vi "Bed_control.vi"(8 "Motor speed":string(combo)="Full step", 9 "pulse duration (T/2)":dbl=0.0005 format="%#_13p", 10 "Sequence to run on start up":string[](array[string]), 11 "Signed pulses to move":dbl=50.0) -> ()   [LabVIEW 2021]
uses:
  <vilib>/DAQmx/write.llb/DAQmx Write (Digital 1D Wfm NChan NSamp).vi
  <vilib>/DAQmx/read.llb/DAQmx Read (Digital 1D Bool 1Chan 1Samp).vi
  <vilib>/Waveform/DWDTOps.llb/DWDT Digital Size.vi
  SmallBore_Labview/global_variables.vi
  <vilib>/DAQmx/create/channels.llb/DAQmx Create Channel (DO-Digital Output).vi
  <vilib>/DAQmx/configure/timing.llb/DAQmx Timing (Sample Clock).vi
  <vilib>/Waveform/DWDTOps.llb/DWDT Uncompress Digital.vi
  <vilib>/DAQmx/miscellaneous.llb/DAQmx Fill In Error Info.vi
  <vilib>/DAQmx/create/channels.llb/DAQmx Create Channel (DI-Digital Input).vi
panel:
  out "data":bool[](array[boolean])
  out "Bed latch switch lines":tag="Dev1/port0/line5:6"
  out "x-y":dbl=626.4
  out "-x":dbl=-24.1
  out "Slide":dbl(slide) min=-35.9 max=609.1 scale=-12.9..637.6
  out "Laser:End dist":dbl=626.4
  out "Home:End dist":dbl=650.5
  out "Home:Laser dist":dbl=24.1
  in  "Save Home-Laser Dist":bool
  in  "Enable Homing Interrupt":bool=TRUE
  in  "Sweep":bool
  out "Main loop has stopped":bool
  out "Last system state called":string="Move"
  in  "Read position":bool
  out "Boolean":bool=TRUE
  in  "Number of runs (>1)":i32=3
  out "Bed position":dbl
  out "Application Directory":path=path "C:/Users/MPI/Documents/GitHub/LabviewGUI"
  out "travel distance (mm)":dbl=5.0
  in  "pulse steps":dbl=50.0 min=0.0 step=1.0 format="%#_6p"
  in  "Move bed 2":bool
  out "Homing in progress":bool
  out "duration of movement":dbl=0.05
  in  "Maximum absolute position":i32=60000 format="%.0p"
  out "Absolute position (pulses)":i32=13150
  in  "Abort movement":bool
  in  "Go home!":bool
  in  "Move bed":bool
  in  "Halt":bool
  # "For programatical use only!\nEnsure that the sequence control is empty before setting default values!"
  # "Step 1: Initiate Homing\nStep 2: Physically press ZERO button\nStep 3: Read position\nStep 4: Go to laser position\nStep 5: Read position\nStep 6: Save current position = Laser\nStep 7: Physically press ZERO button"
  # "Homing"
  # "Enables PDU automatically"
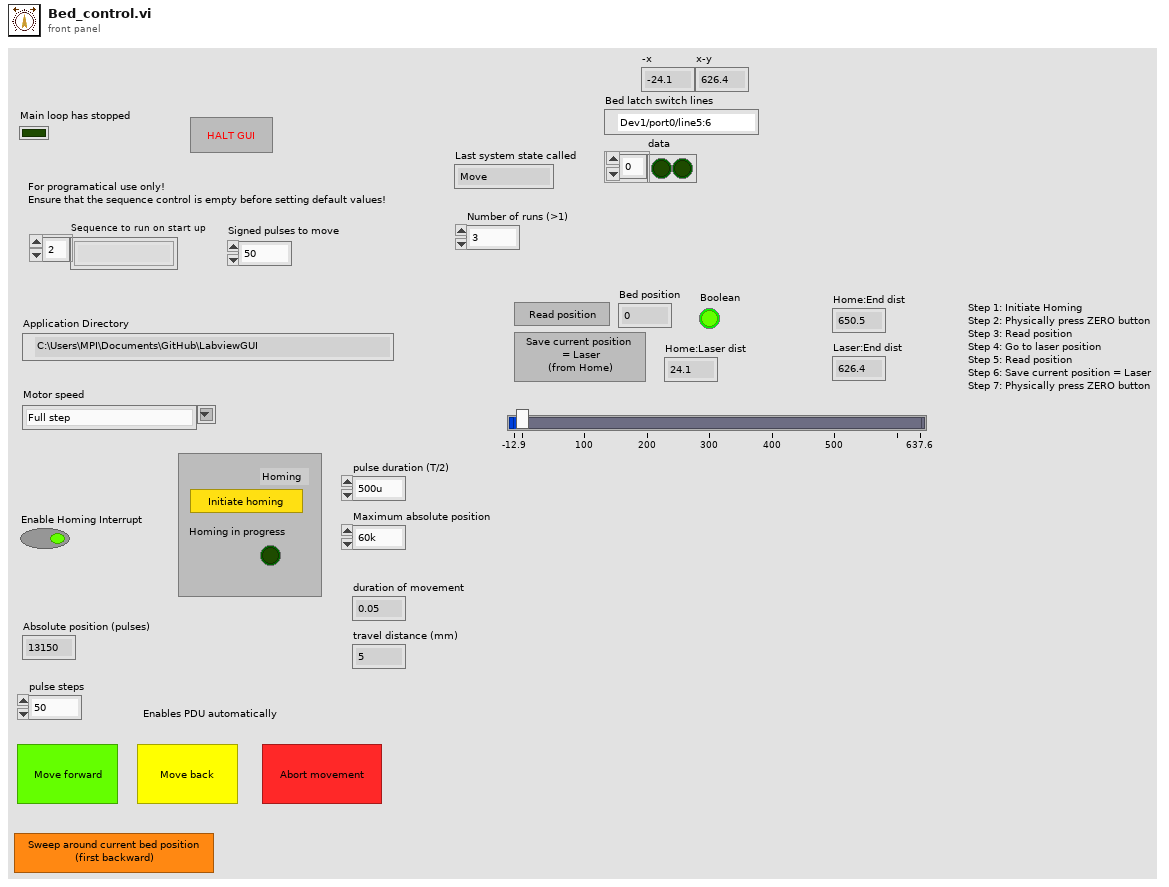
[diagram p1: front panel]
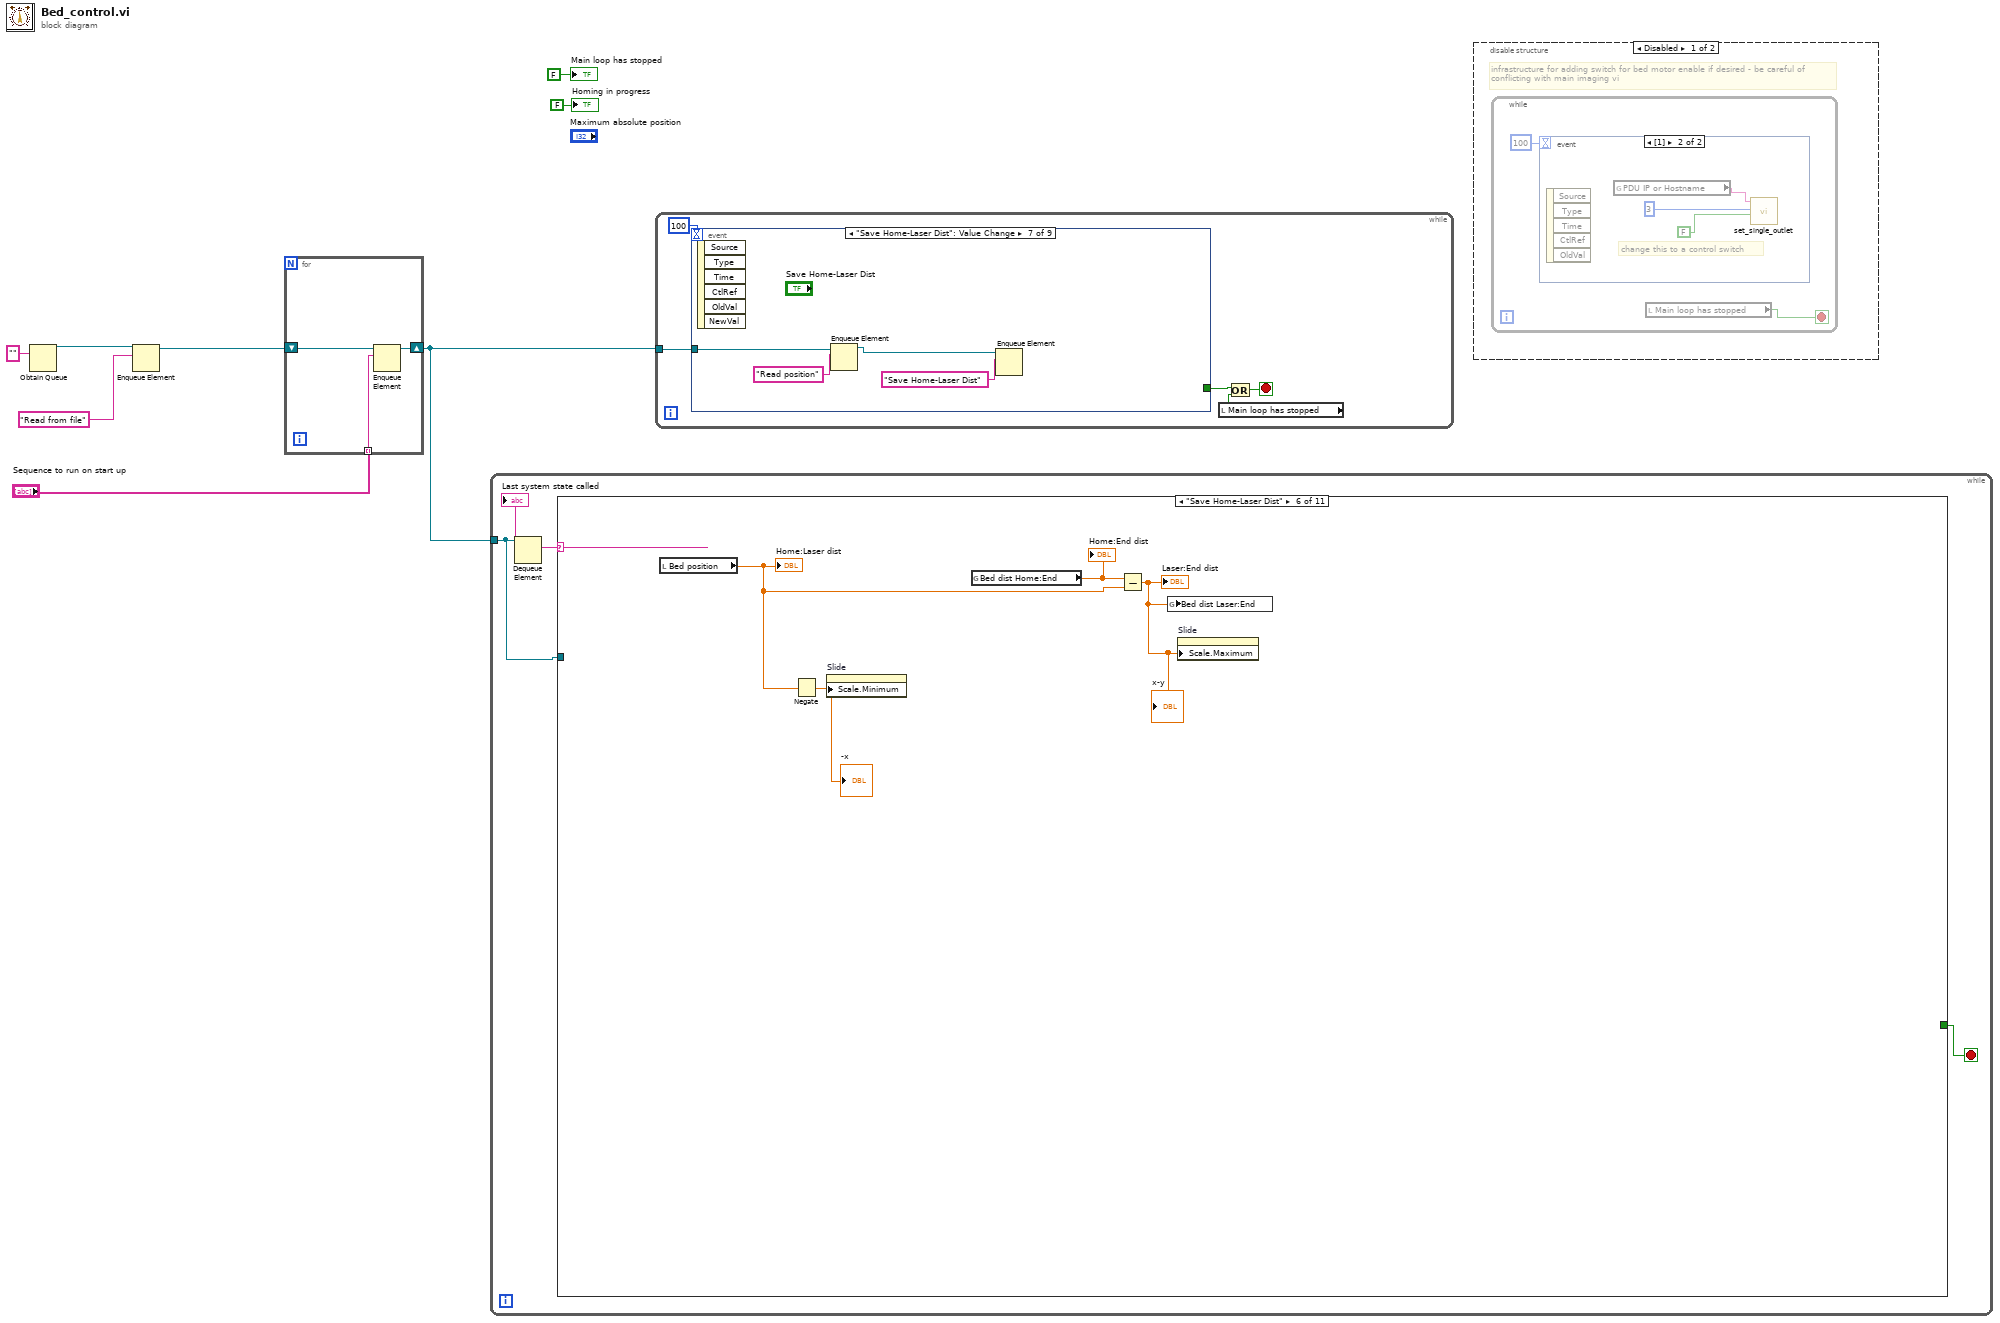
[diagram p0: block diagram]
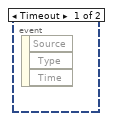
[diagram p2: hidden frame]
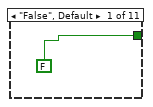
[diagram p4: hidden frame]
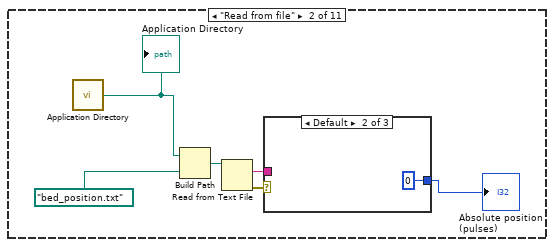
[diagram p5: hidden frame]
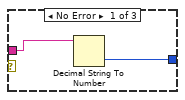
[diagram p6: hidden frame]
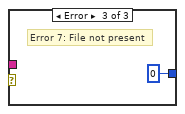
[diagram p7: hidden frame]
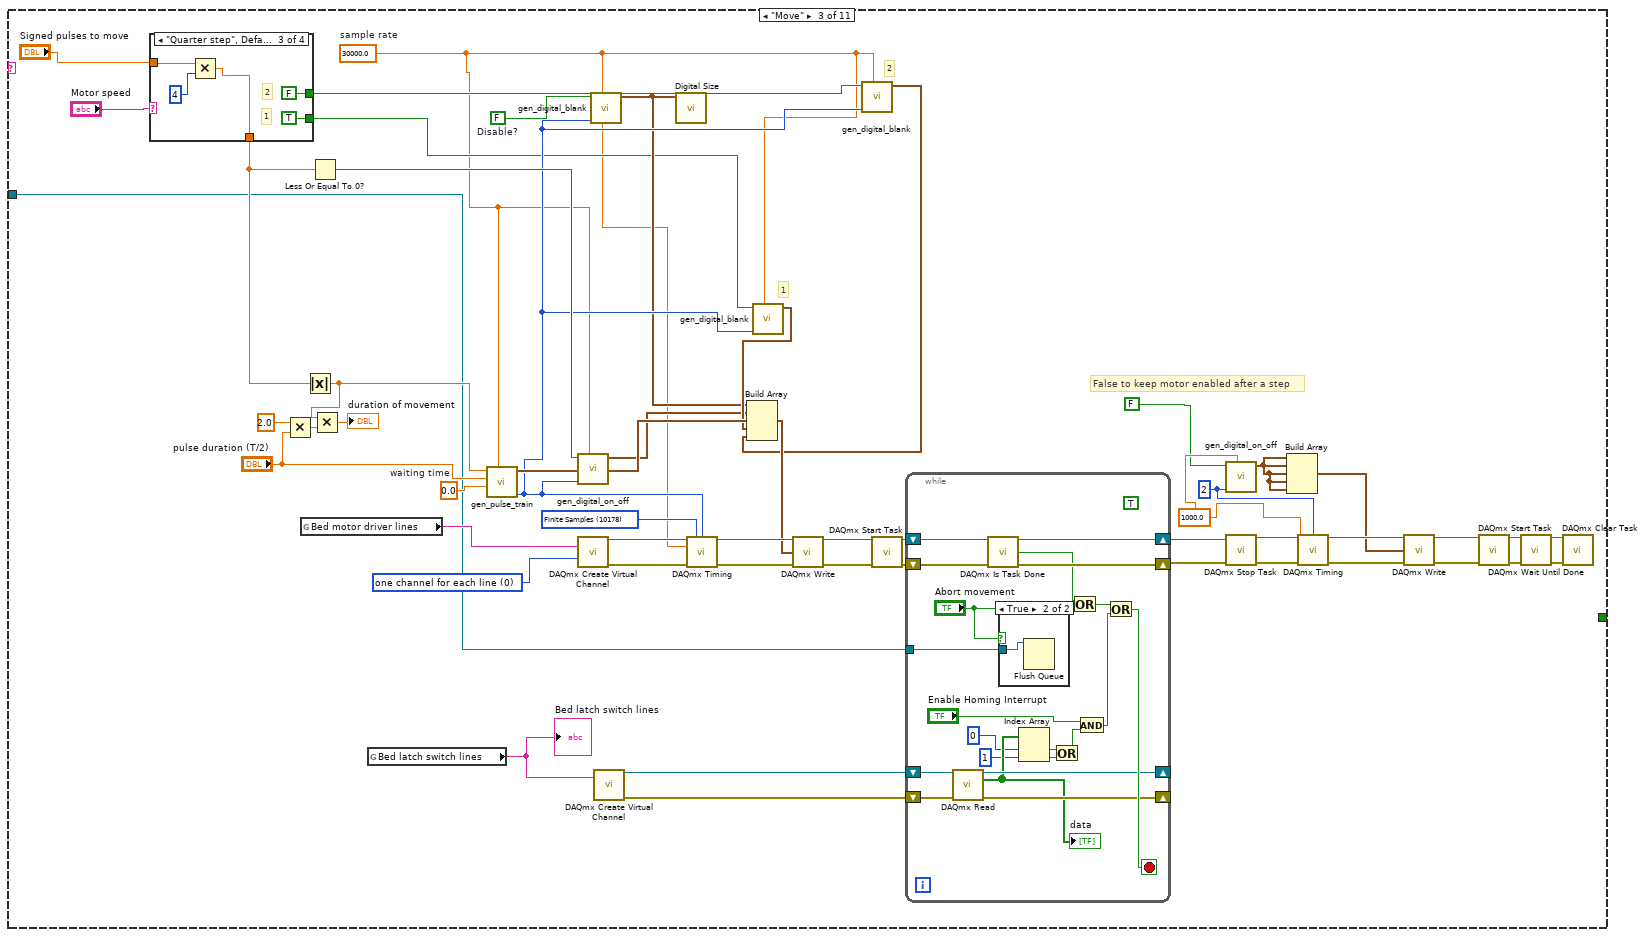
[diagram p8: hidden frame]
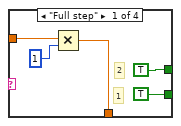
[diagram p9: hidden frame]
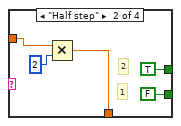
[diagram p10: hidden frame]
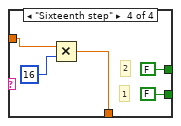
[diagram p11: hidden frame]
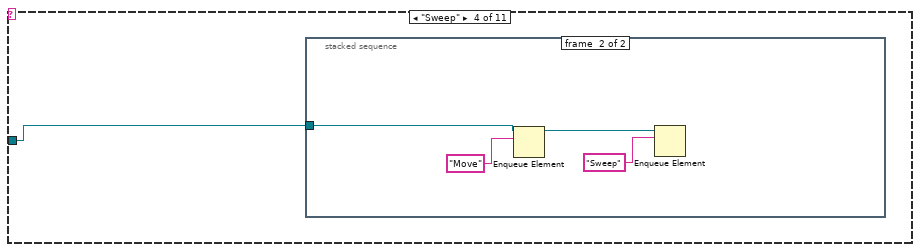
[diagram p13: hidden frame]
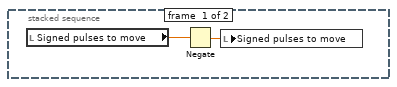
[diagram p14: hidden frame]
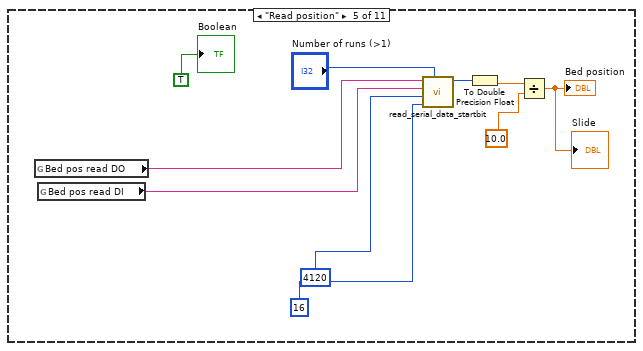
[diagram p15: hidden frame]
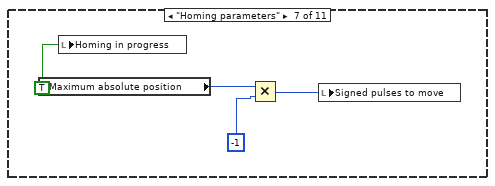
[diagram p16: hidden frame]
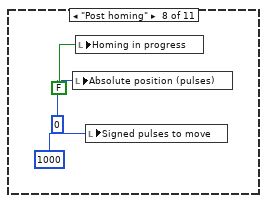
[diagram p17: hidden frame]
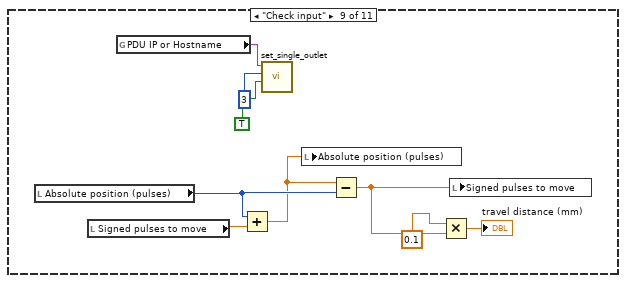
[diagram p18: hidden frame]
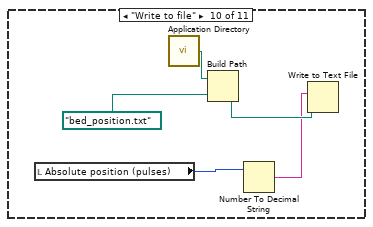
[diagram p19: hidden frame]
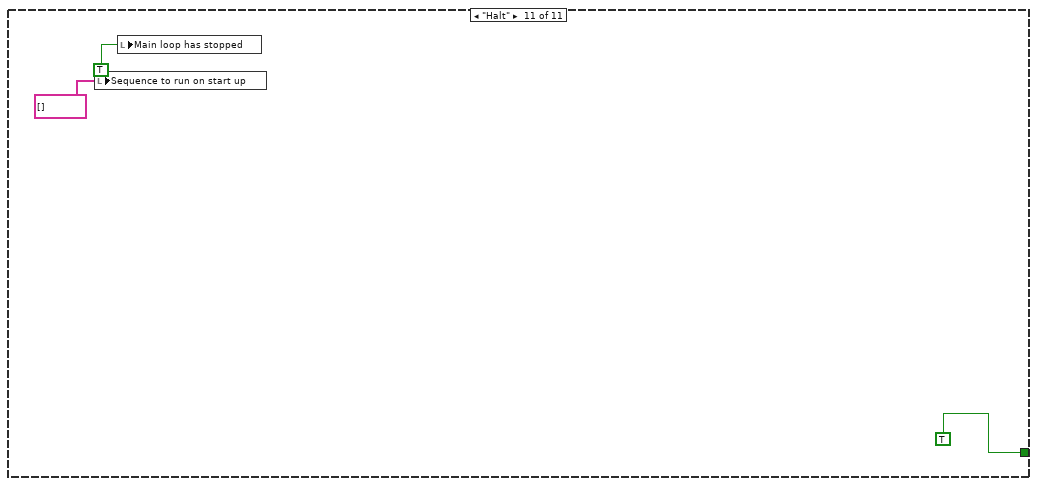
[diagram p20: hidden frame]
diagram:
  n1 = Obtain Queue(element data type="") -> (queue out=w7:refnum<queue>)  [unwired: 4 in, 2 out]
  n2 = Enqueue Element(queue=w7, element="Read from file") -> (queue out=w4:refnum<queue>)  [unwired: 2 in, 2 out]
  n3 = for {
    shift-right: [w10] -> w3
    shift-left: w4 -> [w11]
    tunnel: "Sequence to run on start up" -> [w9] mode=indexing
    n4 = Enqueue Element(queue=w11, element=w9) -> (queue out=w10:refnum<queue>)  [unwired: 2 in, 2 out]
  }
  n5 = while {
    tunnel: w3 -> [w12]
    stop <- w13 stop-if-true
    n6 = Dequeue Element(queue=w12) -> (element=w14:string)  [unwired: 2 in, 3 out]
    "Last system state called" <- w14
    n7 = case shown="\"Save Home-Laser Dist\"" w14 {
      tunnel: [FALSE _ _ _ _ _ _ _ _ _ TRUE] -> w13
      tunnel: w12 -> [_ _ w29 w121 _ _ _ _ _ _ _]
      frame "False", Default {
      }
      frame "Read from file" {
        n8 = call <vilib>:"Application Directory.vi"() -> ("Application Directory"=w18:path)
        "Application Directory" <- w18
        n9 = Build Path(base path=w18, name or relative path=path "bed_position.txt" ("file (use dialog)")) -> (appended path=w19:path)
        n10 = Read from Text File(file (use dialog)=w19) -> (text=w21:string, error out=w20:errorcluster)  [unwired: 3 in, 2 out]
        n11 = case shown="Default" w20 {
          tunnel: w21 -> [w23 _ _]
          tunnel: [w22 0 0] -> w16
          frame No Error {
            n12 = Decimal String To Number(string=w23) -> (number=w22:i32)  [unwired: 2 in, 1 out]
          }
          frame Default {
          }
          frame Error {
            # "Error 7: File not present"
          }
        }
        "Absolute position (pulses)" <- w16
      }
      frame "Move" {
        w45 = 2 ("waveform length")
        w46 = 1000.0 ("rate")
        w68 = 0.0  # waiting time
        w28 = 30000.0  # sample rate
        w71 = FALSE  # Disable?
        w70 = 10178 items=["Finite Samples"=10178, "Continuous Samples"=10123, "Hardware Timed Single Point"=12522] ("sample mode")
        w69 = 0 items=["one channel for each line", "one channel for all lines"] ("line grouping")
        # "1"
        # "2"
        # "False to keep motor enabled after a step"
        n13 = case shown="\"Quarter step\", Default" "Motor speed" {
          tunnel: "Signed pulses to move" -> [w82 w87 w92 w97]
          tunnel: [TRUE ("motor speed control 1") TRUE ("motor speed control 1") FALSE ("motor speed control 1") FALSE ("motor speed control 1")] -> w35
          tunnel: [TRUE ("motor speed control 1") FALSE ("motor speed control 1") TRUE ("motor speed control 1") FALSE ("motor speed control 1")] -> w34
          tunnel: [w79 w84 w89 w94] -> w33
          frame "Full step" {
            # "1"
            # "2"
            n14 = Multiply(x=w82, y=1) -> (x*y=w79:dbl)
          }
          frame "Half step" {
            # "1"
            # "2"
            n15 = Multiply(x=w87, y=2) -> (x*y=w84:dbl)
          }
          frame "Quarter step", Default {
            # "1"
            # "2"
            n16 = Multiply(x=w92, y=4) -> (x*y=w89:dbl)
          }
          frame "Sixteenth step" {
            # "1"
            # "2"
            n17 = Multiply(x=w97, y=16) -> (x*y=w94:dbl)
          }
        }
        n18 = Multiply(x=2.0, y="pulse duration (T/2)") -> (x*y=w64:dbl)
        n19 = global read "global_variables.vi" "Bed motor driver lines"() -> (w32:tag)
        n20 = Absolute Value(x=w33) -> (abs(x)=w65:dbl)
        n21 = Less Or Equal To 0?(x=w33) -> (x <= 0?=w67:bool)
        n22 = Multiply(x=w65, y=w64) -> (x*y=→"duration of movement":dbl)
        n23 = global read "global_variables.vi" "Bed latch switch lines"() -> (w31:tag)
        "Bed latch switch lines" <- w31
        n24 = call "gen_pulse_train.vi"("sampling rate"=w28, "waiting time"=w68, "pulse width"="pulse duration (T/2)", "Number of pulses"=w65) -> ("waveform length"=w42:i32, "digital waveform out"=w76:digitalwaveform)  [unwired: 6 in]
        n25 = call "gen_digital_on_off.vi"("sampling rate"=w28, "waveform length"=w42, "On / Off"=w67) -> ("digital waveform"=w37:digitalwaveform)  [unwired: 8 in]
        n26 = call-poly <vilib>:"DAQmx Create Virtual Channel.vi"("lines"=w32, "line grouping"=w69) -> ("task out"=w72:refnum<k21>, "error out"=w75:errorcluster)  [unwired: 12 in]
        n27 = call "gen_digital_blank.vi"("sampling rate"=w28, "waveform length"=w42, "On / Off"=w71) -> ("digital waveform"=w38:digitalwaveform)  [unwired: 8 in]
        n28 = call-poly <vilib>:"DAQmx Create Virtual Channel.vi"("lines"=w31) -> ("task out"=w27:refnum<k21>, "error out"=w26:errorcluster)  [unwired: 13 in]
        n29 = call-poly <vilib>:"Digital Size.vi"("digital waveform in"=w38) -> ()  [unwired: 7 in, 4 out]
        n30 = call-poly <vilib>:"DAQmx Timing.vi"("task/channels in"=w72, "sample mode"=w70, "samples per channel"=w42, "rate"=w28, "error in"=w75) -> ("task out"=w73:refnum<k21>, "error out"=w74:errorcluster)  [unwired: 9 in]
        n31 = call "gen_digital_blank.vi"("sampling rate"=w28, "waveform length"=w42, "On / Off"=w34) -> ("digital waveform"=w39:digitalwaveform)  [unwired: 8 in]
        n32 = call "gen_digital_blank.vi"("sampling rate"=w28, "waveform length"=w42, "On / Off"=w35) -> ("digital waveform"=w40:digitalwaveform)  [unwired: 8 in]
        n33 = Build Array(w38, w37, w76, w39, w40) -> (w44:digitalwaveform[])
        n34 = call-poly <vilib>:"DAQmx Write.vi"("task/channels in"=w73, "data"=w44, "error in"=w74) -> ("task out"=w77:refnum<k21>, "error out"=w78:errorcluster)  [unwired: 10 in, 1 out]
        n35 = call <vilib>:"DAQmx Start Task.vi"("task/channels in"=w77, "error in"=w78) -> ("task out"=w61:refnum<k21>, "error out"=w60:errorcluster)  [unwired: 12 in]
        n36 = while {
          shift-right: [w116] -> w58
          shift-left: w60 -> [w118]
          shift-right: [w117] -> w59
          shift-left: w61 -> [w119]
          shift-right: [w109] -> _
          shift-left: w27 -> [w112]
          shift-right: [w110] -> _
          shift-left: w26 -> [w111]
          tunnel: w29 -> [w107]
          stop <- w113 stop-if-true
          (unwired) TRUE ("Abort movement")
          n37 = call-poly <vilib>:"DAQmx Read.vi"("task/channels in"=w112, "error in"=w111) -> ("task out"=w109:refnum<k21>, "data"=w104:bool[], "error out"=w110:errorcluster)  [unwired: 11 in]
          "data" <- w104
          n38 = call <vilib>:"DAQmx Is Task Done.vi"("task/channels in"=w119, "error in"=w118) -> ("task out"=w117:refnum<k21>, "task done?"=w115:bool, "error out"=w116:errorcluster)  [unwired: 11 in]
          n39 = case shown="True" "Abort movement" {
            tunnel: w107 -> [_ w120]
            frame False {
            }
            frame True {
              n40 = Flush Queue(queue=w120) -> ()  [unwired: 1 in, 3 out]
            }
          }
          n41 = Index Array(array=w104, index #1=0 ("index"), index #2=1 ("index")) -> (element #1=w100:bool, element #2=w99:bool)
          n42 = Or(x=w100, y=w99) -> (x .or. y?=w101:bool)
          n43 = Or(x=w115, y="Abort movement") -> (x .or. y?=w114:bool)
          n44 = And(x="Enable Homing Interrupt", y=w101) -> (x .and. y?=w105:bool)
          n45 = Or(x=w114, y=w105) -> (x .or. y?=w113:bool)
        }
        n46 = call "gen_digital_on_off.vi"("sampling rate"=w46, "waveform length"=w45, "On / Off"=FALSE ("Keep enabled\n(inverted logic)")) -> ("digital waveform"=w41:digitalwaveform)  [unwired: 8 in]
        n47 = call <vilib>:"DAQmx Stop Task.vi"("task/channels in"=w59, "error in"=w58) -> ("task out"=w48:refnum<k21>, "error out"=w51:errorcluster)  [unwired: 12 in]
        n48 = Build Array(w41, w41, w41, w41, w41) -> (w47:digitalwaveform[])
        n49 = call-poly <vilib>:"DAQmx Timing.vi"("task/channels in"=w48, "samples per channel"=w45, "rate"=w46, "error in"=w51) -> ("task out"=w49:refnum<k21>, "error out"=w50:errorcluster)  [unwired: 10 in]
        n50 = call-poly <vilib>:"DAQmx Write.vi"("task/channels in"=w49, "data"=w47, "error in"=w50) -> ("task out"=w57:refnum<k21>, "error out"=w56:errorcluster)  [unwired: 10 in, 1 out]
        n51 = call <vilib>:"DAQmx Start Task.vi"("task/channels in"=w57, "error in"=w56) -> ("task out"=w55:refnum<k21>, "error out"=w54:errorcluster)  [unwired: 12 in]
        n52 = call <vilib>:"DAQmx Wait Until Done.vi"("task/channels in"=w55, "error in"=w54) -> ("task out"=w53:refnum<k21>, "error out"=w52:errorcluster)  [unwired: 12 in]
        n53 = call <vilib>:"DAQmx Clear Task.vi"("task in"=w53, "error in"=w52) -> ()  [unwired: 13 in, 1 out]
      }
      frame "Sweep" {
        n54 = stacked-sequence {
          tunnel: w121 -> [_ w126]
          frame #0 {
            n55 = local read "Signed pulses to move"() -> (w123:dbl)
            n56 = Negate(x=w123) -> (-x=w122:dbl)
            n57 = local write "Signed pulses to move"(w122) -> ()
          }
          frame #1 {
            n58 = Enqueue Element(queue=w126, element="Move") -> (queue out=w124:refnum<queue>)  [unwired: 2 in, 2 out]
            n59 = Enqueue Element(queue=w124, element="Sweep") -> ()  [unwired: 2 in, 3 out]
          }
        }
      }
      frame "Read position" {
        n60 = global read "global_variables.vi" "Bed pos read DO"() -> (w132:tag)
        n61 = global read "global_variables.vi" "Bed pos read DI"() -> (w131:tag)
        n62 = call "read_serial_data_startbit.vi"("Number of runs"="Number of runs (>1)", "No. expected bits"=u16 16, "baud rate"=u32 4120, "Digital input line"=w131, "Digital output line"=w132) -> ("mode"=w137:i16)  [unwired: 4 in, 1 out]
        n63 = To Double Precision Float(number=w137) -> (double precision float=w135:dbl)
        n64 = Divide(x=w135, y=10.0) -> (x/y=→"Bed position" →"Slide":dbl)
        "Boolean" <- TRUE ("Boolean")
      }
      frame "Save Home-Laser Dist" {
        n65 = local read "Bed position"() -> (w140:dbl)
        "Home:Laser dist" <- w140
        n66 = Negate(x=w140) -> (-x=w139:dbl)
        "-x" <- w139
        n67 = property on="Slide" class="Slide (strict)"("Scale.Minimum"=w139) -> ()  [unwired: 2 in, 2 out]
        n68 = global read "global_variables.vi" "Bed dist Home:End"() -> (w141:dbl)
        "Home:End dist" <- w141
        n69 = Subtract(x=w141, y=w140) -> (x-y=w138:dbl)
        "Laser:End dist" <- w138
        "x-y" <- w138
        n70 = global write "global_variables.vi" "Bed dist Laser:End"(w138) -> ()
        n71 = property on="Slide" class="Slide (strict)"("Scale.Maximum"=w138) -> ()  [unwired: 2 in, 2 out]
      }
      frame "Homing parameters" {
        n72 = local read "Maximum absolute position"() -> (w144:i32)
        n73 = local write "Homing in progress"(TRUE ("Homing in progress")) -> ()
        n74 = Multiply(x=w144, y=-1) -> (x*y=w142:i32)
        n75 = local write "Signed pulses to move"(w142) -> ()
      }
      frame "Post homing" {
        n76 = local write "Absolute position (pulses)"(0 ("Absolute position (pulses)")) -> ()
        n77 = local write "Homing in progress"(FALSE ("Homing in progress")) -> ()
        n78 = local write "Signed pulses to move"(1000 ("pulses to move")) -> ()
      }
      frame "Check input" {
        n79 = local read "Absolute position (pulses)"() -> (w157:i32)
        n80 = local read "Signed pulses to move"() -> (w150:dbl)
        n81 = global read "global_variables.vi" "PDU IP or Hostname"() -> (w153:string)
        n82 = Add(x=w157, y=w150) -> (x+y=w149:dbl)
        n83 = call "set_single_outlet.vi"("Switch state"=TRUE, "Outlet #"=3, "IP / Hostname"=w153) -> ()  [unwired: 9 in]
        n84 = local write "Absolute position (pulses)"(w149) -> ()
        n85 = Subtract(x=w149, y=w157) -> (x-y=w154:dbl)
        n86 = Multiply(x=0.1, y=w154) -> (x*y=→"travel distance (mm)":dbl)
        n87 = local write "Signed pulses to move"(w154) -> ()
      }
      frame "Write to file" {
        n88 = local read "Absolute position (pulses)"() -> (w158:i32)
        n89 = call <vilib>:"Application Directory.vi"() -> ("Application Directory"=w162:path)
        n90 = Build Path(base path=w162, name or relative path=path "bed_position.txt" ("file (use dialog)")) -> (appended path=w161:path)
        n91 = Number To Decimal String(number=w158) -> (decimal integer string=w160:string)  [unwired: 1 in]
        n92 = Write to Text File(file (use dialog)=w161, text=w160) -> ()  [unwired: 2 in, 3 out]
      }
      frame "Halt" {
        n93 = local write "Sequence to run on start up"(string[] [] ("Sequence to run on start up")) -> ()
        n94 = local write "Main loop has stopped"(TRUE ("Main loop has stopped")) -> ()
      }
    }
  }
  n95 = while {
    tunnel: w3 -> [w170]
    stop <- w167 stop-if-true
    n96 = event shown="[6] \"Save Home-Laser Dist\": Value Change" {
      selector: _ -> [_ _ _ _ _ _ _ _ _]
      dyn-events: _ -> [_ _ _ _ _ _ _ _ _]
      timeout: 100 -> [_ _ _ _ _ _ _ _ _]
      tunnel: w170 -> [_ w174 w175 w181 _ w185 w194 w201 w204]
      tunnel: [FALSE TRUE _ _ _ _ _ _ _] -> w168
      event Timeout {
        n97 = event-data() -> ()  [unwired: 1 in, 3 out]
      }
      event "Halt": Value Change {
        n98 = event-data() -> ()  [unwired: 1 in, 6 out]
        n99 = Enqueue Element(queue=w174, element="Halt") -> ()  [unwired: 2 in, 3 out]
      }
      event "Move bed": Value Change {
        n100 = event-data() -> ()  [unwired: 1 in, 6 out]
        n101 = stacked-sequence {
          tunnel: w175 -> [_ w177]
          frame #0 {
            n102 = local write "Signed pulses to move"("pulse steps") -> ()
          }
          frame #1 {
            n103 = Enqueue Element(queue=w177, element="Check input") -> (queue out=w178:refnum<queue>)  [unwired: 2 in, 2 out]
            n104 = Enqueue Element(queue=w178, element="Move") -> ()  [unwired: 2 in, 3 out]
          }
        }
      }
      event "Sweep": Value Change {
        n105 = event-data() -> ()  [unwired: 1 in, 6 out]
        n106 = stacked-sequence {
          tunnel: w181 -> [_ w183]
          frame #0 {
            n107 = local read "pulse steps"() -> (w182:dbl)
            n108 = local write "Signed pulses to move"(w182) -> ()
          }
          frame #1 {
            n109 = Enqueue Element(queue=w183, element="Sweep") -> ()  [unwired: 2 in, 3 out]
          }
        }
      }
      event Key Down? {
        n110 = event-data() -> ()  [unwired: 1 in, 10 out]
        n111 = event-data() -> ()  [unwired: 7 in, 1 out]
      }
      event "Move bed 2": Value Change {
        n112 = event-data() -> ()  [unwired: 1 in, 6 out]
        n113 = stacked-sequence {
          tunnel: w185 -> [_ w188]
          frame #0 {
            n114 = local read "pulse steps"() -> (w186:dbl)
            n115 = Negate(x=w186) -> (-x=w187:dbl)
            n116 = local write "Signed pulses to move"(w187) -> ()
          }
          frame #1 {
            n117 = Enqueue Element(queue=w188, element="Check input") -> (queue out=w189:refnum<queue>)  [unwired: 2 in, 2 out]
            n118 = Enqueue Element(queue=w189, element="Move") -> ()  [unwired: 2 in, 3 out]
          }
        }
      }
      event "Save Home-Laser Dist": Value Change {
        n119 = event-data() -> ()  [unwired: 1 in, 6 out]
        n120 = Enqueue Element(queue=w194, element="Read position") -> (queue out=w192:refnum<queue>)  [unwired: 2 in, 2 out]
        n121 = Enqueue Element(queue=w192, element="Save Home-Laser Dist") -> ()  [unwired: 2 in, 3 out]
      }
      event "Go home!": Value Change {
        n122 = event-data() -> ()  [unwired: 1 in, 6 out]
        n123 = local write "Enable Homing Interrupt"("Go home!") -> ()
        n124 = Enqueue Element(queue=w201, element="Homing parameters") -> (queue out=w199:refnum<queue>)  [unwired: 2 in, 2 out]
        n125 = Enqueue Element(queue=w199, element="Move") -> (queue out=w197:refnum<queue>)  [unwired: 2 in, 2 out]
        n126 = Enqueue Element(queue=w197, element="Post homing") -> ()  [unwired: 2 in, 3 out]
      }
      event "Read position": Value Change {
        n127 = event-data() -> ()  [unwired: 1 in, 6 out]
        n128 = Enqueue Element(queue=w204, element="Read position") -> ()  [unwired: 2 in, 3 out]
      }
    }
    n129 = local read "Main loop has stopped"() -> (w169:bool)
    n130 = Or(x=w168, y=w169) -> (x .or. y?=w167:bool)
  }
  n131 = disable-structure shown="Disabled" {
    frame Disabled {
      # "infrastructure for adding switch for bed motor enable if desired - be careful of conflicting with main imaging vi"
      n132 = while {
        stop <- w205 stop-if-true
        n133 = event shown="[1]" {
          selector: _ -> [_ _]
          dyn-events: _ -> [_ _]
          timeout: 100 -> [_ _]
          event Timeout {
            n134 = event-data() -> ()  [unwired: 1 in, 3 out]
          }
          event #1 (no event record) {
            # "change this to a control switch"
            n135 = event-data() -> ()  [unwired: 1 in, 5 out]
            n136 = global read "global_variables.vi" "PDU IP or Hostname"() -> (w209:string)
            n137 = call "set_single_outlet.vi"("Switch state"=FALSE, "Outlet #"=3, "IP / Hostname"=w209) -> ()  [unwired: 9 in]
          }
        }
        n138 = local read "Main loop has stopped"() -> (w205:bool)
      }
    }
    frame Enabled {
    }
  }
  "Homing in progress" <- FALSE ("Homing in progress")
  "Main loop has stopped" <- FALSE ("Main loop has stopped")
